vi "Get Thread Reference.vi"(8 "error in (no error)":errorcluster, 11 "WebSocket in":refnum<class "WebSocket.lvclass">) -> (0 "error out":errorcluster, 1 "Thread VI":refnum<vi>, 3 "WebSocket out":refnum<class "WebSocket.lvclass">)   [LabVIEW 2017, in "WebSocket.lvclass"]
uses:
  WebSocket.lvclass
  Thread.vi
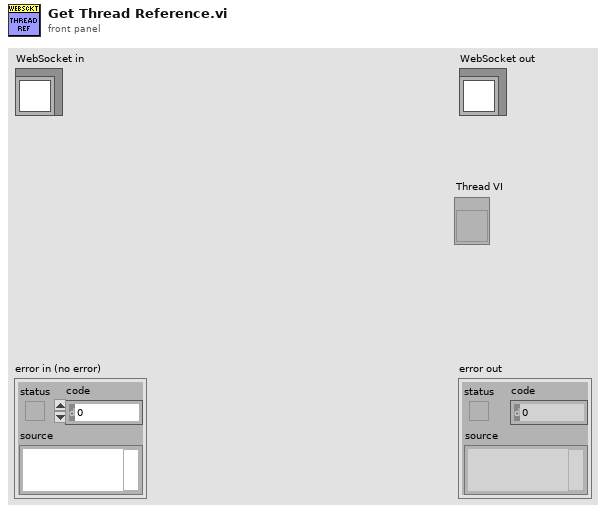
[diagram p1: front panel]
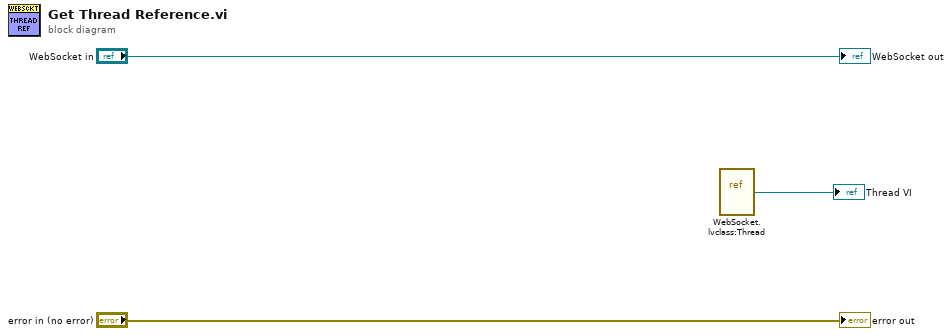
[diagram p0: block diagram]
diagram:
  n1 = vi-ref "WebSocket.lvclass:Thread.vi"() -> (→"Thread VI":refnum<vi>)
  "error out" <- "error in (no error)"
  "WebSocket out" <- "WebSocket in"
